vi "Serialize - JSON.vi"(8 "error in":errorcluster, 11 "xData in":refnum<class "xData.lvclass">) -> (0 "error out":errorcluster, 2 "Serialized JSON":string, 3 "xData out":refnum<class "xData.lvclass">)   [LabVIEW 2014, in "xData.lvclass"]
uses:
  xData.lvclass
  reusable/Data/Data.lvclass/Data.ctl
  xData.lvclass/xData.ctl
  reusable/Data/Write write time.vi
  reusable/Data/Data.lvclass
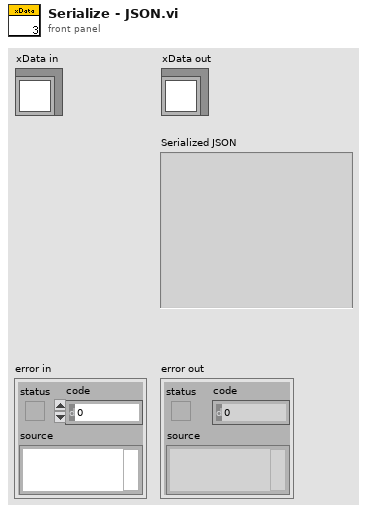
[diagram p1: front panel]
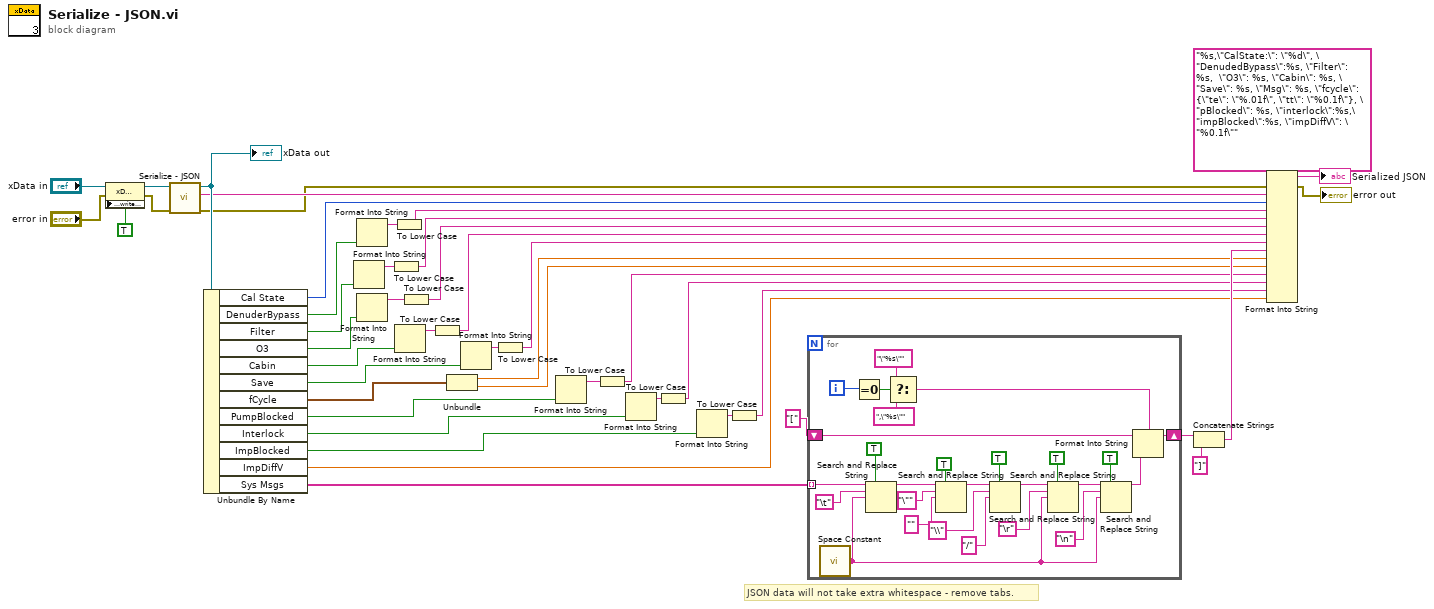
[diagram p0: block diagram]
diagram:
  # "JSON data will not take extra whitespace - remove tabs."
  n1 = property class="xData"(reference="xData in", error in="error in", "Accessors:write time"=TRUE ("write time")) -> (reference out=w26:refnum<class "xData.lvclass">, error out=w7:errorcluster)
  n2 = call-parent "Serialize - JSON.vi"("error in"=w7, "Data in"=w26) -> ("error out"=w30:errorcluster, "Serialized JSON"=w43:string, "Data out"=w45:refnum<class "xData.lvclass">)  [unwired: 7 in]
  "xData out" <- w45
  n3 = Unbundle By Name(w45) -> ("Cal State"=w1:u8, "DenuderBypass"=w2:bool, "Filter"=w41:bool, "O3"=w39:bool, "Cabin"=w36:bool, "Save"=w32:bool, "fCycle"=w21:cluster{"telapsed":dbl, "ttotal":sgl}, "PumpBlocked"=w17:bool, "Interlock"=w13:bool, "ImpBlocked"=w10:bool, "ImpDiffV"=w18:dbl, "Sys Msgs"=w6:string[])
  n4 = Format Into String(w41) -> (resulting string=w4:string)  [unwired: 3 in, 1 out]
  n5 = Format Into String(w2) -> (resulting string=w5:string)  [unwired: 3 in, 1 out]
  n6 = Format Into String(w39) -> (resulting string=w38:string)  [unwired: 3 in, 1 out]
  n7 = To Lower Case(string=w4) -> (all lower case string=w40:string)
  n8 = To Lower Case(string=w5) -> (all lower case string=w3:string)
  n9 = Format Into String(w36) -> (resulting string=w35:string)  [unwired: 3 in, 1 out]
  n10 = To Lower Case(string=w38) -> (all lower case string=w37:string)
  n11 = To Lower Case(string=w35) -> (all lower case string=w34:string)
  n12 = Unbundle(w21) -> ("telapsed"=w20:dbl, "ttotal"=w19:sgl)
  n13 = Format Into String(w32) -> (resulting string=w33:string)  [unwired: 3 in, 1 out]
  n14 = To Lower Case(string=w33) -> (all lower case string=w31:string)
  n15 = Format Into String(w17) -> (resulting string=w16:string)  [unwired: 3 in, 1 out]
  n16 = To Lower Case(string=w16) -> (all lower case string=w15:string)
  n17 = Format Into String(w13) -> (resulting string=w14:string)  [unwired: 3 in, 1 out]
  n18 = To Lower Case(string=w14) -> (all lower case string=w12:string)
  n19 = Format Into String(w10) -> (resulting string=w11:string)  [unwired: 3 in, 1 out]
  n20 = To Lower Case(string=w11) -> (all lower case string=w9:string)
  n21 = for {
    tunnel: w6 -> [w64] mode=indexing
    shift-right: [w70] -> w24
    shift-left: "[" -> [w71]
    i -> [w68]
    n22 = call <vilib>:"Space Constant.vi"() -> ("String"=w47:string)
    n23 = Equal To 0?(x=w68) -> (x = 0?=w69:bool)
    n24 = Search and Replace String(replace all?=TRUE ("replace all? (F)"), input string=w64, search string="\t", replace string=w47) -> (result string=w60:string)  [unwired: 4 in, 3 out]
    n25 = Select(t="\"%s\"", s=w69, f=",\"%s\"") -> (s? t:f=w65:string)
    n26 = Search and Replace String(replace all?=TRUE ("replace all? (F)"), input string=w60, search string="\"", replace string="" ("replace string (\"\")")) -> (result string=w57:string)  [unwired: 4 in, 3 out]
    n27 = Search and Replace String(replace all?=TRUE ("replace all? (F)"), input string=w57, search string="\\", replace string="/" ("replace string (\"\")")) -> (result string=w51:string)  [unwired: 4 in, 3 out]
    n28 = Search and Replace String(replace all?=TRUE ("replace all? (F)"), input string=w51, search string="\r", replace string=w47) -> (result string=w50:string)  [unwired: 4 in, 3 out]
    n29 = Search and Replace String(replace all?=TRUE ("replace all? (F)"), input string=w50, search string="\n", replace string=w47) -> (result string=w49:string)  [unwired: 4 in, 3 out]
    n30 = Format Into String(format string=w65, initial string=w71, w49) -> (resulting string=w70:string)  [unwired: 1 in, 1 out]
  }
  n31 = Concatenate Strings(w24, "]" ("string")) -> (w22:string)
  n32 = Format Into String(format string="%s,\"CalState:\": \"%d\", \"DenudedBypass\":%s, \"Filter\": %s,  \"O3\": %s, \"Cabin\": %s, \"Save\": %s, \"Msg\": %s, \"fcycle\": {\"te\": \"%.01f\", \"tt\": \"%0.1f\"}, \"pBlocked\": %s, \"interlock\":%s,\"impBlocked\":%s, \"impDiffV\": \"%0.1f\"", error in=w30, w43, w1, w3, w40, w37, w34, w31, w22, w20, w19, w15, w12, w9, w18) -> (resulting string=→"Serialized JSON":string, error out=→"error out":errorcluster)  [unwired: 1 in]
